vi "Update EXE Icons.vi"(8 "error in (no error)":errorcluster, 10 "ICO Paths":path[](array[path]), 11 "EXE Path":path) -> (0 "error out":errorcluster)   [LabVIEW 2011]
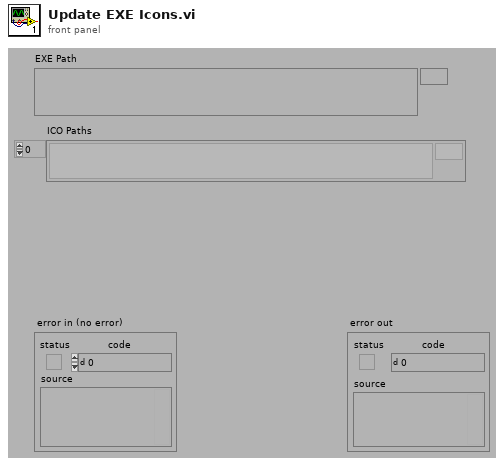
[diagram p1: front panel]
types:
  T1 = typedef "IconInfo.ctl" = cluster{"Width":u8, "Height":u8, "Depth":u8, "Resource Data":u8[]}
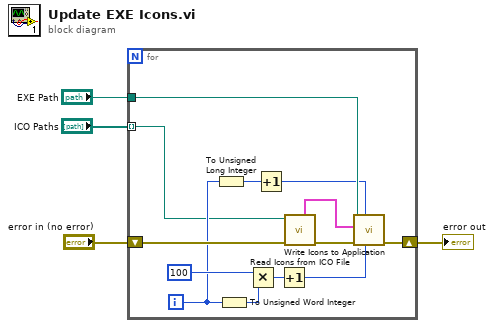
[diagram p0: block diagram]
diagram:
  n1 = for {
    tunnel: "EXE Path" -> [w15]
    shift-right: [w6] -> w2
    shift-left: "error in (no error)" -> [w14]
    tunnel: "ICO Paths" -> [w5] mode=indexing
    i -> [w8]
    n2 = To Unsigned Long Integer(number=w8) -> (unsigned 32bit integer=w7:u32)
    n3 = To Unsigned Word Integer(number=w8) -> (unsigned 16bit integer=w10:u16)
    n4 = Multiply(x=u16 100 ("Base Icon ID (for subimages)"), y=w10) -> (x*y=w12:u16)
    n5 = Increment(x=w7) -> (x+1=w9:u32)
    n6 = Increment(x=w12) -> (x+1=w11:u16)
    n7 = call <vilib>:"Read Icons from ICO File.vi"("error in (no error)"=w14, "file path"=w5) -> ("error out"=w16:errorcluster, "Icon Info"=w17:T1[])  [unwired: 1 in, 7 out]
    n8 = call <vilib>:"Write Icons to Application.vi"("Base Icon ID (for subimages)"=w11, "iconID (for group)"=w9, "error in"=w16, "Icon Infos"=w17, "Path to Exe"=w15) -> ("error out"=w6:errorcluster)  [unwired: 6 out]
  }
  "error out" <- w2
